vi "Config_test.vi"() -> ()   [LabVIEW 2020]
uses:
  <vilib>/Utility/config.llb/Read Key (String).vi
  <vilib>/Utility/config.llb/NI_LVConfig.lvlib
panel:
  out "output cluster":T1 {"MaxCurrent [A]" format="%.2f"; "StabilitySetting [%]" format="%.2f"; "FieldCurrentRatio [T/A]" format="%.2f"; "SwitchWaitTime [s]" format="%.2f"; "SwitchHtrCurrent [mA]" format="%.2f"; "TrainRates [T]" format="%.2f"; "NormalRates [T]" format="%.2f"; "Breakpts [A]" format="%.2f"}
  in  "Input Cluster":T1 {"MaxCurrent [A]" format="%.2f"; "StabilitySetting [%]" format="%.2f"; "FieldCurrentRatio [T/A]" format="%.2f"; "SwitchWaitTime [s]" format="%.2f"; "SwitchHtrCurrent [mA]" format="%.2f"; "TrainRates [T]" format="%.5e"; "NormalRates [T]" format="%.5e"; "Breakpts [A]" format="%.5e"}
  out "message":string=" INSTRUCTIONS:\r\rNormal Use:  When using subVIs that incorporate the error in/error out (or error I/O) structure, place this handler where you want to inform the user of an error, typically at the end of the I/O data path, as the last action of the program.  If the error in error? is ERROR, the handler creates a message describing the error and its source.  If the type of dialog = 1 (default), the message is displayed to the user, who can only acknowedge it.  If the type = 2, the user can acknowledge the message or abort execution; aborting a program with active I/O is not recommended.  If the type = 0, no message is displayed; this is used to process the error programmatically, and the error out cluster elements are wired to individual terminals for that reason.  \r\rOther Use:\n\r\nlocal testing.  To test the error code of a subVI or function that does not have the error I/O structure, you can wire its error code and a source string to the local error code and error source inputs.  If error in error? indicates no error and error code is not equal to 0, the local code and source are substituted for the error in values, and error? is set TRUE (ERROR)."
  in  "error in (no error)":errorcluster
  out "error out":errorcluster
  out "key names":string[](array[string])
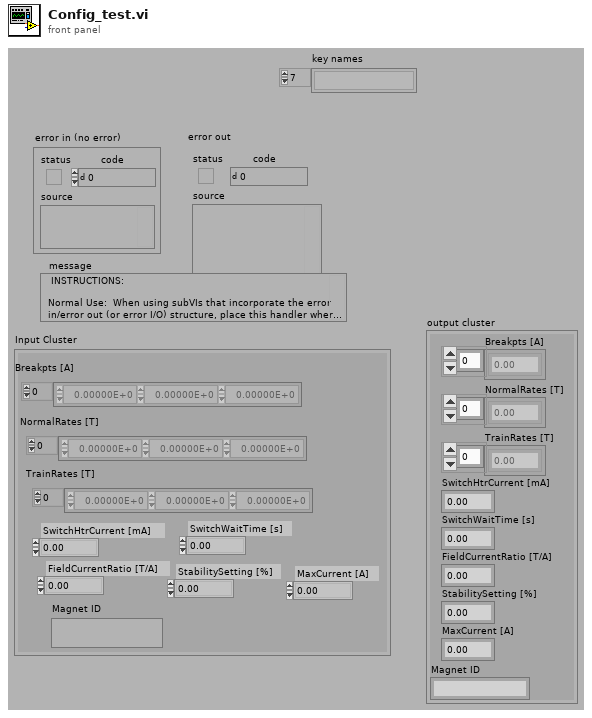
[diagram p1: front panel]
types:
  T1 = cluster{"Breakpts [A]":dbl[], "NormalRates [T]":dbl[], "TrainRates [T]":dbl[], "SwitchHtrCurrent [mA]":dbl, "SwitchWaitTime [s]":dbl, "FieldCurrentRatio [T/A]":dbl, "StabilitySetting [%]":dbl, "MaxCurrent [A]":dbl, "Magnet ID":string}
  T2 = typedef "NI_LVConfig.lvlib/Config Data RefNum.ctl" = refnum<k1>
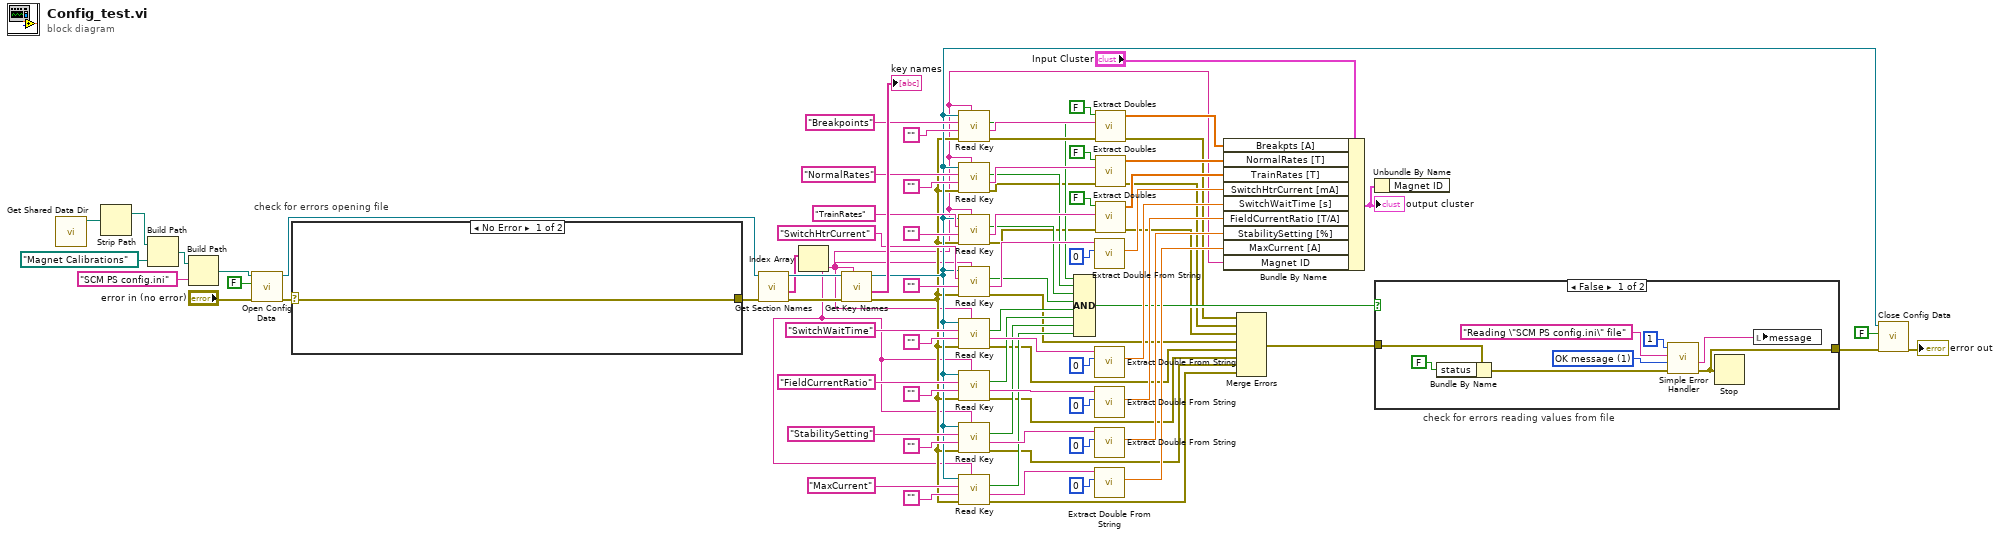
[diagram p0: block diagram]
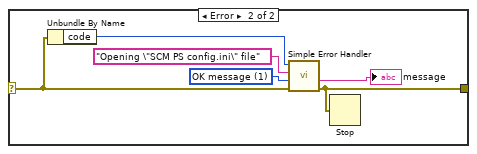
[diagram p3: hidden frame]
diagram:
  # "check for errors reading values from file"
  # "check for errors opening file"
  n1 = call "Get Shared Data Dir.vi"() -> ("Data Directory Path"=w8:path)  [unwired: 2 in, 1 out]
  n2 = Strip Path(path=w8) -> (stripped path=w9:path)  [unwired: 1 out]
  n3 = Build Path(base path=w9, name or relative path=path "Magnet Calibrations") -> (appended path=w80:path)
  n4 = Build Path(base path=w80, name or relative path="SCM PS config.ini") -> (appended path=w81:path)
  n5 = call <vilib>:"Open Config Data.vi"("error in (no error)"="error in (no error)", "create file if necessary (T)"=FALSE ("create file if necessary? (T)"), "configuration file path"=w81) -> ("error out"=w10:errorcluster, "refnum"=w5:T2)  [unwired: 6 in, 1 out]
  n6 = case shown="No Error" w10 {
    selector: w10 -> [w85 w86]
    tunnel: [w85 w88] -> w6
    frame No Error {
    }
    frame Error {
      w89 = u16 1 items=["no dialog", "OK message", "continue or stop message"] ("type of dialog (OK msg:1)")
      n7 = Unbundle By Name(w86) -> ("code"=w87:i32)
      n8 = call <vilib>:"Simple Error Handler.vi"("error code (no error:0)"=w87, "error source (\" \")"="Opening \"SCM PS config.ini\" file" ("error source (\" \")"), "type of dialog (OK msg:1)"=w89, "error in (no error)"=w86) -> ("source out"=→"message":string, "error out"=w88:errorcluster)  [unwired: 1 in, 3 out]
      n9 = Stop(stop? (T)=w88) -> ()
    }
  }
  n10 = call <vilib>:"Get Section Names.vi"("error in (no error)"=w6, "refnum"=w5) -> ("error out"=w3:errorcluster, "section names"=w1:string[], "refnum out"=w4:T2)  [unwired: 7 in]
  n11 = Index Array(array=w1) -> (element=w2:string)  [unwired: 1 in]
  n12 = call <vilib>:"Get Key Names.vi"("section"=w2, "error in (no error)"=w3, "refnum"=w4) -> ("error out"=w20:errorcluster, "key names"=→"key names":string[], "refnum out"=w45:T2)  [unwired: 5 in, 1 out]
  n13 = call-poly <vilib>:"Read Key.vi"("section"=w2, "error in (no error)"=w20, "default value"="", "key"="Breakpoints", "refnum"=w45) -> ("error out"=w32:errorcluster, "value"=w74:string, "found?"=w31:bool)  [unwired: 3 in, 1 out]
  n14 = call-poly <vilib>:"Read Key.vi"("section"=w2, "error in (no error)"=w20, "default value"="", "key"="NormalRates", "refnum"=w45) -> ("error out"=w22:errorcluster, "value"=w70:string, "found?"=w30:bool)  [unwired: 3 in, 1 out]
  n15 = call-poly <vilib>:"Read Key.vi"("section"=w2, "error in (no error)"=w20, "default value"="", "key"="TrainRates", "refnum"=w45) -> ("error out"=w21:errorcluster, "value"=w66:string, "found?"=w29:bool)  [unwired: 3 in, 1 out]
  n16 = call-poly <vilib>:"Read Key.vi"("section"=w2, "error in (no error)"=w20, "default value"="", "key"="SwitchHtrCurrent", "refnum"=w45) -> ("error out"=w15:errorcluster, "value"=w62:string, "found?"=w28:bool)  [unwired: 3 in, 1 out]
  n17 = call-poly <vilib>:"Read Key.vi"("section"=w2, "error in (no error)"=w20, "default value"="", "key"="SwitchWaitTime", "refnum"=w45) -> ("error out"=w14:errorcluster, "value"=w58:string, "found?"=w27:bool)  [unwired: 3 in, 1 out]
  n18 = call-poly <vilib>:"Read Key.vi"("section"=w2, "error in (no error)"=w20, "default value"="", "key"="FieldCurrentRatio", "refnum"=w45) -> ("error out"=w13:errorcluster, "value"=w54:string, "found?"=w26:bool)  [unwired: 3 in, 1 out]
  n19 = call-poly <vilib>:"Read Key.vi"("section"=w2, "error in (no error)"=w20, "default value"="", "key"="StabilitySetting", "refnum"=w45) -> ("error out"=w12:errorcluster, "value"=w50:string, "found?"=w25:bool)  [unwired: 3 in, 1 out]
  n20 = call-poly <vilib>:"Read Key.vi"("section"=w2, "error in (no error)"=w20, "default value"="", "key"="MaxCurrent", "refnum"=w45) -> ("error out"=w11:errorcluster, "value"=w46:string, "found?"=w24:bool)  [unwired: 3 in, 1 out]
  n21 = Compound Arithmetic op=AND(w31, w30, w29, w28, w27, w26, w25, w24) -> (w23:bool)
  n22 = call "Extract Double From String.vi"("start index"=0, "string"=w62) -> ("floating pt. number"=w39:dbl)  [unwired: 2 in, 3 out]
  n23 = call "Extract Double From String.vi"("start index"=0, "string"=w58) -> ("floating pt. number"=w38:dbl)  [unwired: 2 in, 3 out]
  n24 = call "Extract Double From String.vi"("start index"=0, "string"=w54) -> ("floating pt. number"=w37:dbl)  [unwired: 2 in, 3 out]
  n25 = call "Extract Double From String.vi"("start index"=0, "string"=w50) -> ("floating pt. number"=w36:dbl)  [unwired: 2 in, 3 out]
  n26 = call "Extract Double From String.vi"("start index"=0, "string"=w46) -> ("floating pt. number"=w35:dbl)  [unwired: 2 in, 3 out]
  n27 = call "Extract Doubles.vi"("error in"=w32, "String"=w74, "Eng Units?"=FALSE) -> ("error out"=w18:errorcluster, "Data"=w43:dbl[])  [unwired: 3 in]
  n28 = call "Extract Doubles.vi"("error in"=w22, "String"=w70, "Eng Units?"=FALSE) -> ("error out"=w17:errorcluster, "Data"=w41:dbl[])  [unwired: 3 in]
  n29 = call "Extract Doubles.vi"("error in"=w21, "String"=w66, "Eng Units?"=FALSE) -> ("error out"=w16:errorcluster, "Data"=w40:dbl[])  [unwired: 3 in]
  n30 = Bundle By Name(cluster="Input Cluster", "Breakpts [A]"=w43, "NormalRates [T]"=w41, "TrainRates [T]"=w40, "SwitchHtrCurrent [mA]"=w39, "SwitchWaitTime [s]"=w38, "FieldCurrentRatio [T/A]"=w37, "StabilitySetting [%]"=w36, "MaxCurrent [A]"=w35, "Magnet ID"=w2) -> (w34:T1)
  "output cluster" <- w34
  n31 = Merge Errors(w18, w17, w16, w15, w14, w13, w12, w11) -> (w19:errorcluster)
  n32 = Unbundle By Name(w34) -> ()  [unwired: 1 out]
  n33 = case shown="False" w23 {
    tunnel: [w93 w100] -> w44
    tunnel: w19 -> [w96 w100]
    frame False {
      w98 = u16 1 items=["no dialog", "OK message", "continue or stop message"] ("type of dialog (OK msg:1)")
      n34 = Bundle By Name(cluster=w96, "status"=FALSE) -> (w94:errorcluster)
      n35 = call <vilib>:"Simple Error Handler.vi"("error code (no error:0)"=1, "error source (\" \")"="Reading \"SCM PS config.ini\" file" ("error source (\" \")"), "type of dialog (OK msg:1)"=w98, "error in (no error)"=w94) -> ("source out"=w97:string, "error out"=w93:errorcluster)  [unwired: 1 in, 3 out]
      n36 = Stop(stop? (T)=w93) -> ()
      n37 = local write "message"(w97) -> ()
    }
    frame True {
    }
  }
  n38 = call <vilib>:"Close Config Data.vi"("error in (no error)"=w44, "write file if changed (T)"=FALSE ("write configuration file? (T)"), "refnum"=w45) -> ("error out"=→"error out":errorcluster)  [unwired: 7 in, 1 out]
